vi "Nested Core.vi"(8 "error in (no error)":errorcluster, 10 "key":string, 11 "JSON Value in":refnum<class "JSON Value.lvclass">) -> (0 "error out":errorcluster, 2 "stop?":bool, 3 "JSON Value out":refnum<class "JSON Value.lvclass">)   [LabVIEW 2016, in "JSON Value.lvclass"]
uses:
  JSON Value.lvclass
  Errors.ctl
  Object/Get Value/Get Value (Value).vi
  Array/Index Array/Index Array (Value).vi
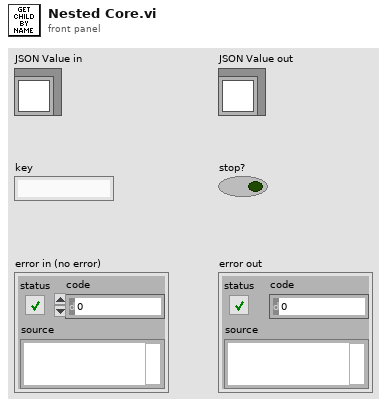
[diagram p1: front panel]
types:
  T1 = typedef "JSON Value.lvclass/JSON Types.ctl" = enum8{"String", "Numeric", "Boolean", "NULL", "Object", "Array"}
  T2 = typedef "JSON Value.lvclass/Errors.ctl" = enum8{"No key", "Key path type", "Array OOB", "Type Mismatch", "Invalid Token"}
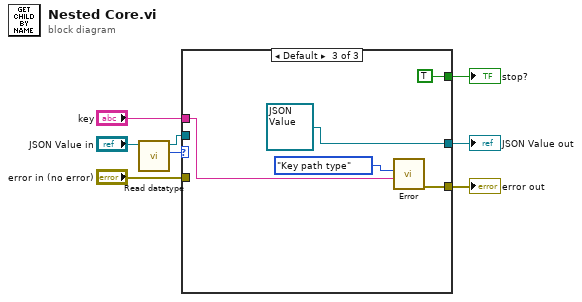
[diagram p0: block diagram]
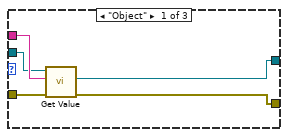
[diagram p2: hidden frame]
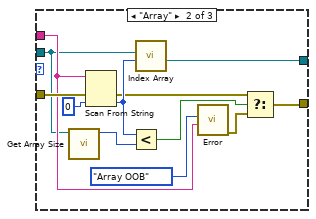
[diagram p3: hidden frame]
diagram:
  n1 = call "Read datatype.vi"("JSON Value in"="JSON Value in") -> ("datatype"=w2:T1, "JSON Value out"=w1:refnum<class "JSON Value.lvclass">)  [unwired: 8 in, 1 out]
  n2 = case shown="Default" w2 {
    tunnel: "key" -> [w12 w15 w27]
    tunnel: [w11 w24 refnum<class "JSON Value.lvclass"> refnum ("JSON Object in")] -> w8
    tunnel: w1 -> [w9 w14 _]
    tunnel: [w10 w17 w29] -> w5
    tunnel: "error in (no error)" -> [w13 w23 _]
    tunnel: [_ _ TRUE] -> w7
    frame "Object" {
      n3 = call-poly "Get Value.vi"("error in (no error)"=w13, "key"=w12, "JSON Value in"=w9) -> ("error out"=w10:errorcluster, "JSON Value out"=w11:refnum<class "JSON Value.lvclass">)  [unwired: 7 in]
    }
    frame "Array" {
      n4 = call "Get Array Size.vi"("JSON Value in"=w14) -> ("size(s)"=w22:i32)  [unwired: 9 in, 1 out]
      n5 = Scan From String(input string=w15, error in=w23, default 1=0 ("index")) -> (error out=w19:errorcluster, output 1=w21:i32)  [unwired: 2 in, 2 out]
      n6 = Less?(x=w21, y=w22) -> (x < y?=w20:bool)
      n7 = call-poly "Index Array.vi"("index"=w21, "JSON Value in"=w14) -> ("JSON Value out"=w24:refnum<class "JSON Value.lvclass">)  [unwired: 8 in, 1 out]
      n8 = call "Error.vi"("Data"=w15, "Error"=Errors."Array OOB") -> ("error out"=w18:errorcluster)  [unwired: 8 in]
      n9 = Select(t=w19, s=w20, f=w18) -> (s? t:f=w17:errorcluster)
    }
    frame Default {
      n10 = call "Error.vi"("Data"=w27, "Error"=Errors."Key path type") -> ("error out"=w29:errorcluster)  [unwired: 8 in]
    }
  }
  "JSON Value out" <- w8
  "stop?" <- w7
  "error out" <- w5
